vi "Scan SysCfg Device Information.vi"(6 "Expose System Hardware Reference":bool, 8 "error in":errorcluster, 11 "Refnum in":refnum<k21>) -> (0 "error out":errorcluster, 2 "Network Device":T1 {"Product ID" format="%.0x"; "Primary Network Adapter"."IP Address Request Mode" items=["Static"=1, "DHCP/Link Local"=2, "Link-Local Only"=4, "DHCP Only"=8]; "Primary Network Adapter"."Adapter Type" items=["Ethernet"=1, "WLAN"=2]; "Primary Network Adapter"."Adapter Mode" items=["Disabled"=1, "TCP/IP Ethernet"=2, "Deterministic"=4, "EtherCAT"=8, "TCP/IP WLAN Connect"=32, "TCP/IP WLAN Create"=64]; "Secondary Network Adapters"."IP Address Request Mode" items=["Static"=1, "DHCP/Link Local"=2, "Link-Local Only"=4, "DHCP Only"=8]; "Secondary Network Adapters"."Adapter Type" items=["Disabled"=1, "TCP/IP Ethernet"=2, "Deterministic"=4, "EtherCAT"=8, "TCP/IP WLAN Connect"=32, "TCP/IP WLAN Create"=64]; "Secondary Network Adapters"."Adapter Mode" items=["Disabled"=1, "TCP/IP Ethernet"=2, "Deterministic"=4, "EtherCAT"=8, "TCP/IP WLAN Connect"=32, "TCP/IP WLAN Create"=64]}, 3 "Refnum out":refnum<k21>)   [LabVIEW 2015, in "SMI.lvlib" / "Controller.lvclass"]
uses:
  Controller.lvclass
  Controls/ControllerInformation.ctl
  Controls/DeviceInformation.ctl
  Controls/NetworkAdapterSettings.ctl
  <vilib>/nisyscfg/Close (Filter).vi
  <vilib>/nisyscfg/Close (Resources).vi
  <vilib>/nisyscfg/Find Hardware.vi
  <resource>/objmgr/niflexriosae.rc
  <vilib>/nisyscfg/nisyscfg.lvlib
  <resource>/objmgr/nisysapi.rc
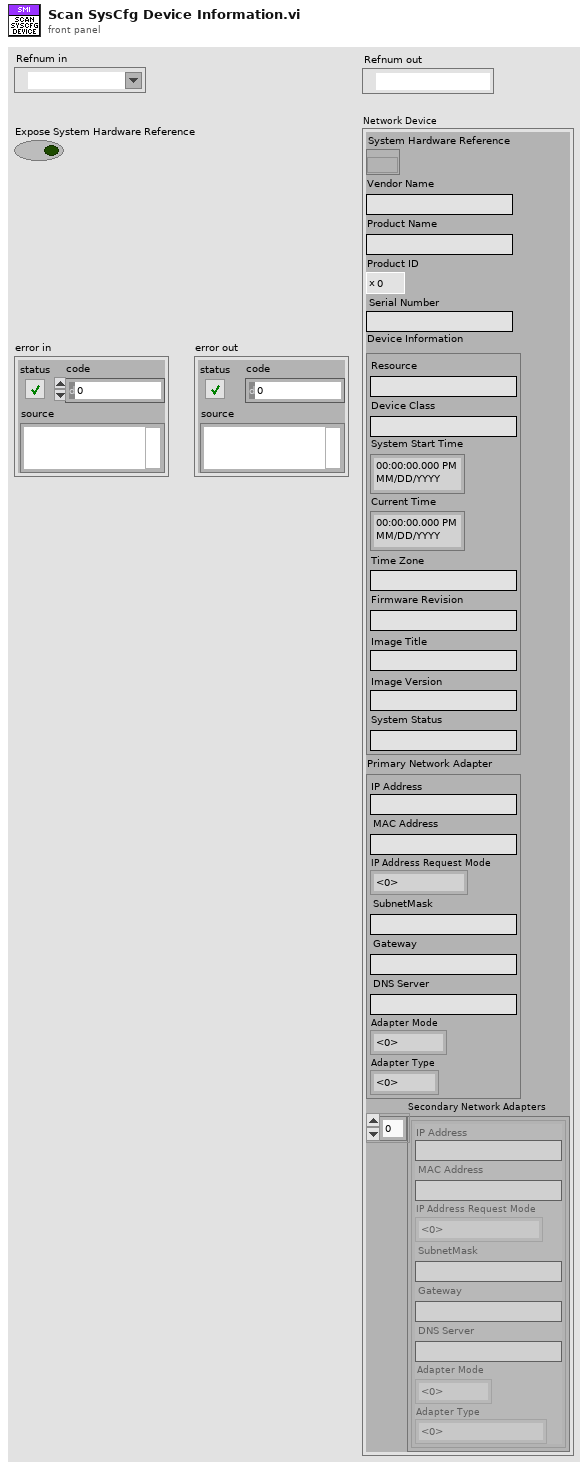
[diagram p1: front panel]
types:
  T1 = typedef "SMI.lvlib/Controller.lvclass/ControllerInformation.ctl" = cluster{"System Hardware Reference":refnum<k20>, "Vendor Name":string, "Product Name":string, "Product ID":u16, "Serial Number":string, "Device Information":T2, "Primary Network Adapter":T3, "Secondary Network Adapters":T3[]}
  T2 = typedef "SMI.lvlib/Controller.lvclass/DeviceInformation.ctl" = cluster{"Resource":string, "Device Class":string, "System Start Time":timestamp, "Current Time":timestamp, "Time Zone":string, "Firmware Revision":string, "Image Title":string, "Image Version":string, "System Status":string}
  T3 = typedef "SMI.lvlib/Controller.lvclass/NetworkAdapterSettings.ctl" = cluster{"IP Address":string, "MAC Address":string, "IP Address Request Mode":u32, "SubnetMask":string, "Gateway":string, "DNS Server":string, "Adapter Mode":u32, "Adapter Type":u32}
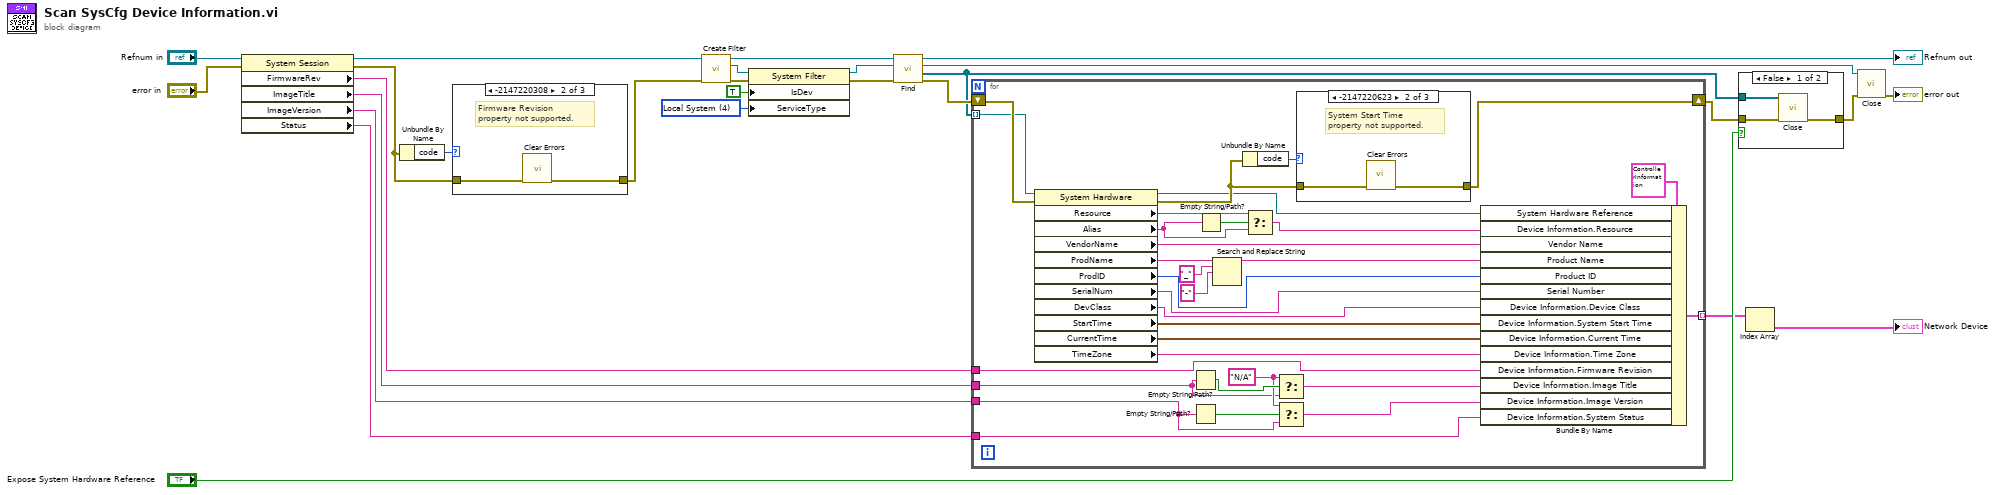
[diagram p0: block diagram]
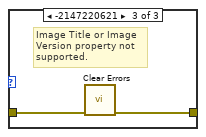
[diagram p3: hidden frame]
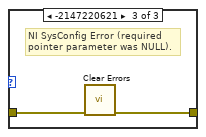
[diagram p6: hidden frame]
diagram:
  w25 = u32 4 items=["NI Network Resource", "NI Real-Time", "NI System Configuration", "NI Web Interface", "Local System", "Local Network Adapter", "Local Time Keeper", "Local Time Reference", "LXI Instrument", "Local FPGA"] ("Service Type")
  n1 = property class="System Session"(reference="Refnum in", error in="error in") -> (reference out=w21:refnum<k21>, error out=w2:errorcluster, "FirmwareRev"=w12:string, "ImageTitle"=w7:string, "ImageVersion"=w5:string, "Status"=w6:string)
  n2 = Unbundle By Name(w2) -> ("code"=w1:i32)
  n3 = case shown="-2147220308" w1 {
    tunnel: w2 -> [w28 w30 w32]
    tunnel: [w28 w29 w31] -> w20
    frame Default {
    }
    frame -2147220308 {
      # "Firmware Revision\nproperty not supported."
      n4 = call <vilib>:"Clear Errors.vi"("error in (no error)"=w30) -> ("error out"=w29:errorcluster)  [unwired: 5 in, 1 out]
    }
    frame -2147220621 {
      # "Image Title or Image\nVersion property not \nsupported."
      n5 = call <vilib>:"Clear Errors.vi"("error in (no error)"=w32) -> ("error out"=w31:errorcluster)  [unwired: 5 in, 1 out]
    }
  }
  n6 = call <vilib>:"Create Filter.vi"("error in (no error)"=w20, "Session in"=w21) -> ("error out"=w17:errorcluster, "Filter out"=w18:refnum<k20>, "Session out"=w22:refnum<k21>)  [unwired: 7 in]
  n7 = property class="System Filter"(reference=w18, error in=w17, "IsDev"=TRUE ("Is Device"), "ServiceType"=w25) -> (reference out=w23:refnum<k20>, error out=w19:errorcluster)
  n8 = call-poly <vilib>:"Find.vi"("error in (no error)"=w19, "Filter in"=w23, "Session in"=w22) -> ("error out"=w13:errorcluster, "Resources out"=w10:refnum<k20>[], "Filter out"=w9:refnum<k20>, "Session out"=→"Refnum out":refnum<k21>)  [unwired: 5 in]
  n9 = for {
    tunnel: w5 -> [w36]
    tunnel: w6 -> [w64]
    tunnel: w7 -> [w35]
    tunnel: w10 -> [w41] mode=indexing
    tunnel: [w59] -> w15 mode=indexing
    tunnel: w12 -> [w58]
    shift-right: [w61] -> w11
    shift-left: w13 -> [w57]
    w37 = "N/A"
    n10 = property class="System Hardware"(reference=w41, error in=w57) -> (reference out=w40:refnum<k20>, error out=w63:errorcluster, "Resource"=w54:string, "Alias"=w53:string, "VendorName"=w50:string, "ProdName"=w48:string, "ProdID"=w45:u32, "SerialNum"=w46:string, "DevClass"=w42:string, "StartTime"=w51:timestamp, "CurrentTime"=w55:timestamp, "TimeZone"=w56:string)
    n11 = Empty String/Path?(string/path=w35) -> (empty?=w38:bool)
    n12 = Empty String/Path?(string/path=w36) -> (empty?=w39:bool)
    n13 = Empty String/Path?(string/path=w53) -> (empty?=w52:bool)
    n14 = Search and Replace String(input string=w48, search string="_", replace string="-" ("replace string (\"\")")) -> (result string=w47:string)  [unwired: 5 in, 3 out]
    n15 = Unbundle By Name(w63) -> ("code"=w62:i32)
    n16 = Select(t=w54, s=w52, f=w53) -> (s? t:f=w49:string)
    n17 = Select(t=w37, s=w38, f=w35) -> (s? t:f=w33:string)
    n18 = Select(t=w37, s=w39, f=w36) -> (s? t:f=w34:string)
    n19 = case shown="-2147220623" w62 {
      tunnel: w63 -> [w65 w67 w69]
      tunnel: [w65 w66 w68] -> w61
      frame Default {
      }
      frame -2147220623 {
        # "System Start Time\nproperty not supported."
        n20 = call <vilib>:"Clear Errors.vi"("error in (no error)"=w67) -> ("error out"=w66:errorcluster)  [unwired: 5 in, 1 out]
      }
      frame -2147220621 {
        # "NI SysConfig Error (required\npointer parameter was NULL)."
        n21 = call <vilib>:"Clear Errors.vi"("error in (no error)"=w69) -> ("error out"=w68:errorcluster)  [unwired: 5 in, 1 out]
      }
    }
    n22 = Bundle By Name(cluster=T1 {"System Hardware Reference"=refnum, "Vendor Name"="", "Product Name"="", "Product ID"=0, "Serial Number"="", "Device Information"={"Resource"="", "Device Class"="", "System Start Time"=timestamp(0 s since 1904-01-01), "Current Time"=timestamp(0 s since 1904-01-01), "Time Zone"="", "Firmware Revision"="", "Image Title"="", "Image Version"="", "System Status"=""}, "Primary Network Adapter"={"IP Address"="", "MAC Address"="", "IP Address Request Mode"=1, "SubnetMask"="", "Gateway"="", "DNS Server"="", "Adapter Mode"=1, "Adapter Type"=1}, "Secondary Network Adapters"=[]} ("Network Device"), "System Hardware Reference"=w40, "Device Information.Resource"=w49, "Vendor Name"=w50, "Product Name"=w47, "Product ID"=w45, "Serial Number"=w46, "Device Information.Device Class"=w42, "Device Information.System Start Time"=w51, "Device Information.Current Time"=w55, "Device Information.Time Zone"=w56, "Device Information.Firmware Revision"=w58, "Device Information.Image Title"=w33, "Device Information.Image Version"=w34, "Device Information.System Status"=w64) -> (w59:T1)
  }
  n23 = case shown="False" "Expose System Hardware Reference" {
    tunnel: [w72 w73] -> w8
    tunnel: w10 -> [w71 _]
    tunnel: w11 -> [w70 w73]
    frame False {
      n24 = call-poly <vilib>:"Close.vi"("error in (no error)"=w70, "Resources in"=w71) -> ("error out"=w72:errorcluster)  [unwired: 9 in]
    }
    frame True {
    }
  }
  n25 = Index Array(array=w15) -> (element=→"Network Device":T1)  [unwired: 1 in]
  n26 = call-poly <vilib>:"Close.vi"("error in (no error)"=w8, "Filter in"=w9) -> ("error out"=→"error out":errorcluster)  [unwired: 9 in]
